vi "Moto_MSB2StBit.vi"(10 "长度":string, 11 "MSB":string) -> (3 "起始位":string)   [LabVIEW 2015]
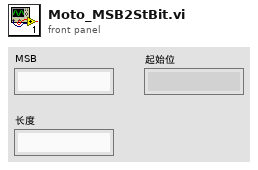
[diagram p1: front panel]
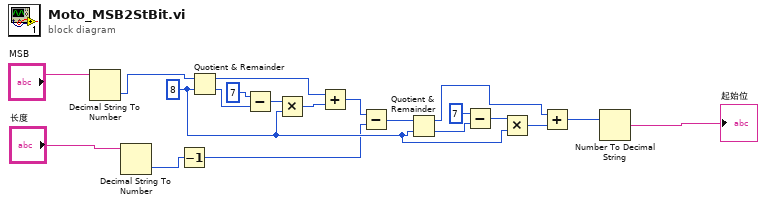
[diagram p0: block diagram]
diagram:
  w16 = 8
  n1 = Decimal String To Number(string="MSB") -> (number=w9:i32)  [unwired: 2 in, 1 out]
  n2 = Decimal String To Number(string="长度") -> (number=w8:i32)  [unwired: 2 in, 1 out]
  n3 = Decrement(x=w8) -> (x-1=w11:i32)
  n4 = Quotient & Remainder(x=w9, y=w16) -> (x-y*floor(x/y)=w2:i32, floor(x/y)=w4:i32)
  n5 = Subtract(x=7, y=w4) -> (x-y=w3:i32)
  n6 = Multiply(x=w3, y=w16) -> (x*y=w5:i32)
  n7 = Add(x=w2, y=w5) -> (x+y=w10:i32)
  n8 = Subtract(x=w10, y=w11) -> (x-y=w12:i32)
  n9 = Quotient & Remainder(x=w12, y=w16) -> (x-y*floor(x/y)=w18:i32, floor(x/y)=w14:i32)
  n10 = Subtract(x=7, y=w14) -> (x-y=w15:i32)
  n11 = Multiply(x=w15, y=w16) -> (x*y=w17:i32)
  n12 = Add(x=w18, y=w17) -> (x+y=w19:i32)
  n13 = Number To Decimal String(number=w19) -> (decimal integer string=→"起始位":string)  [unwired: 1 in]
